vi "Display Contour SPINE Head Tail (SubVI).vi"(0 "Display Data":T1) -> (4 "Contour Array":cluster{"Array":i32[], "Array":i32[]}[](array[cluster]), 6 "SPINE Array":cluster{"Array":i32[], "Array":i32[]}[](array[cluster]), 8 "Head Array":cluster{"Array":i32[], "Array":i32[]}[](array[cluster]), 10 "Tail Array":cluster{"Array":i32[], "Array":i32[]}[](array[cluster]), 15 "Larvae ID":u32[](array[numeric]))   [LabVIEW 2020]
uses:
  Controls (HOST)/Data to Disk Bundle.ctl
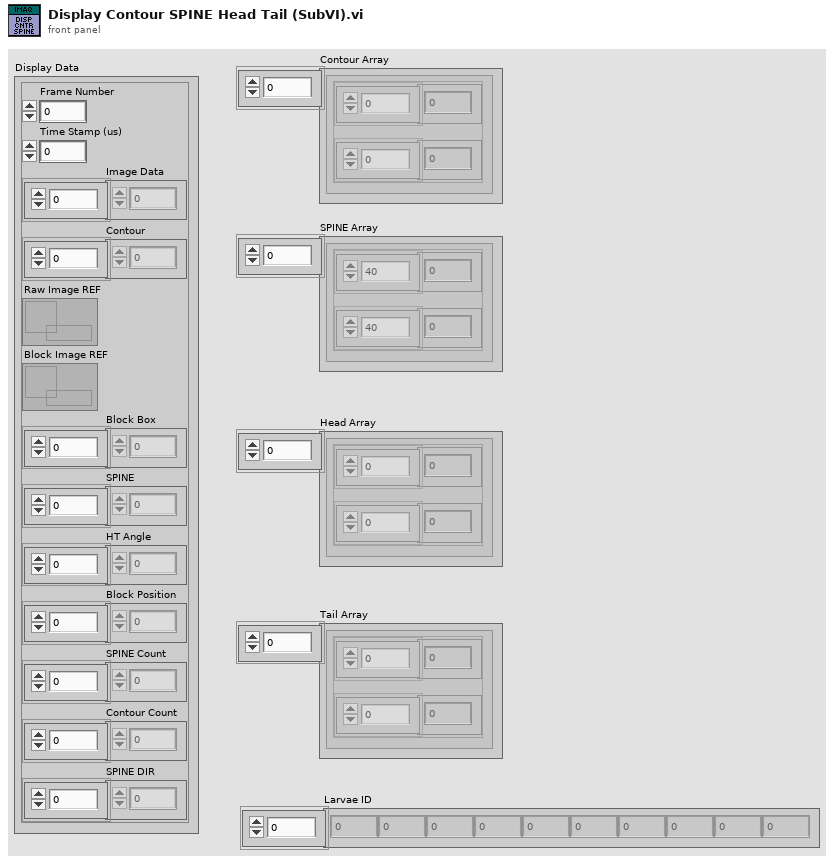
[diagram p1: front panel]
types:
  T1 = typedef "Data to Disk Bundle.ctl" = cluster{"Frame Number":u64, "Time Stamp (us)":u64, "Image Data":u64[], "Contour":u32[], "Raw Image REF":refnum<data-value>, "Block Image REF":refnum<data-value>, "Block Box":u64[], "SPINE":u32[], "HT Angle":u64[], "Block Position":u64[], "SPINE Count":u32[], "Contour Count":u32[], "SPINE DIR":u8[]}
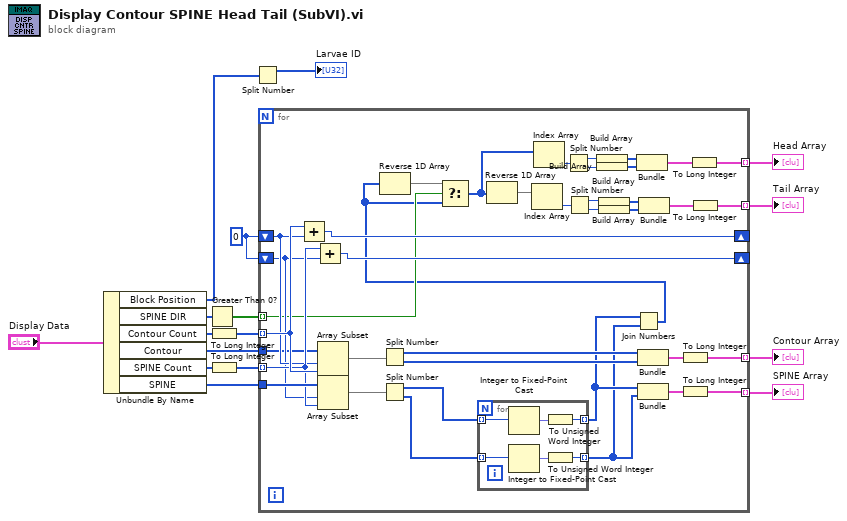
[diagram p0: block diagram]
diagram:
  w14 = 0 ("Numeric Control")
  n1 = Unbundle By Name("Display Data") -> ("Block Position"=w1:u64[], "SPINE DIR"=w3:u8[], "Contour Count"=w9:u32[], "Contour"=w8:u32[], "SPINE Count"=w16:u32[], "SPINE"=w15:u32[])
  n2 = Greater Than 0?(x=w3) -> (x > 0?=w2:bool[])
  n3 = To Long Integer(number=w9) -> (32bit integer=w13:i32[])
  n4 = To Long Integer(number=w16) -> (32bit integer=w12:i32[])
  n5 = Split Number(x=w1) -> (hi(x)=→"Larvae ID":u32[])  [unwired: 1 out]
  n6 = for {
    tunnel: w13 -> [w52] mode=indexing
    tunnel: w8 -> [w39]
    tunnel: w12 -> [w51] mode=indexing
    tunnel: w15 -> [w53]
    shift-right: [w55] -> _
    shift-left: w14 -> [w50]
    shift-right: [w54] -> _
    shift-left: w14 -> [w49]
    tunnel: [w41] -> w10 mode=indexing
    tunnel: [w40] -> w4 mode=indexing
    tunnel: [w25] -> w6 mode=indexing
    tunnel: [w24] -> w5 mode=indexing
    tunnel: w2 -> [w26] mode=indexing
    n7 = Add(x=w52, y=w50) -> (x+y=w55:i32)
    n8 = Add(x=w51, y=w49) -> (x+y=w54:i32)
    n9 = Array Subset(array=w39, index=w50, length=w52) -> (w48:u32[])
    n10 = Array Subset(array=w53, index=w49, length=w51) -> (w27:u32[])
    n11 = Split Number(x=w48) -> (hi(x)=w23:u16[], lo(x)=w22:u16[])
    n12 = Split Number(x=w27) -> (hi(x)=w21:u16[], lo(x)=w20:u16[])
    n13 = for {
      tunnel: w21 -> [w61] mode=indexing
      tunnel: w20 -> [w60] mode=indexing
      tunnel: [w57] -> w19 mode=indexing
      tunnel: [w56] -> w18 mode=indexing
      n14 = Integer to Fixed-Point Cast(integer=w61) -> (fixed-point=w59:fxp<+,16,9>)  [unwired: 1 in]
      n15 = Integer to Fixed-Point Cast(integer=w60) -> (fixed-point=w58:fxp<+,16,9>)  [unwired: 1 in]
      n16 = To Unsigned Word Integer(number=w59) -> (unsigned 16bit integer=w57:u16)
      n17 = To Unsigned Word Integer(number=w58) -> (unsigned 16bit integer=w56:u16)
    }
    n18 = Join Numbers(hi=w19, lo=w18) -> ((hi.lo)=w17:u32[])
    n19 = Reverse 1D Array(array=w17) -> (reversed array=w35:u32[])
    n20 = Select(t=w35, s=w26, f=w17) -> (s? t:f=w36:u32[])
    n21 = Reverse 1D Array(array=w36) -> (reversed array=w32:u32[])
    n22 = Index Array(array=w32) -> (element=w33:u32)  [unwired: 1 in]
    n23 = Index Array(array=w36) -> (element=w34:u32)  [unwired: 1 in]
    n24 = Split Number(x=w34) -> (hi(x)=w28:u16, lo(x)=w29:u16)
    n25 = Split Number(x=w33) -> (hi(x)=w30:u16, lo(x)=w31:u16)
    n26 = Build Array(w28) -> (w45:u16[])
    n27 = Build Array(w29) -> (w44:u16[])
    n28 = Build Array(w30) -> (w42:u16[])
    n29 = Build Array(w31) -> (w43:u16[])
    n30 = Bundle(w45, w44) -> (w37:cluster{u16[], u16[]})  [unwired: 1 in]
    n31 = Bundle(w23, w22) -> (w47:cluster{u16[], u16[]})  [unwired: 1 in]
    n32 = Bundle(w19, w18) -> (w46:cluster{u16[], u16[]})  [unwired: 1 in]
    n33 = Bundle(w42, w43) -> (w38:cluster{u16[], u16[]})  [unwired: 1 in]
    n34 = To Long Integer(number=w47) -> (32bit integer=w41:cluster{i32[], i32[]})
    n35 = To Long Integer(number=w46) -> (32bit integer=w40:cluster{i32[], i32[]})
    n36 = To Long Integer(number=w37) -> (32bit integer=w25:cluster{i32[], i32[]})
    n37 = To Long Integer(number=w38) -> (32bit integer=w24:cluster{i32[], i32[]})
  }
  "Contour Array" <- w10
  "SPINE Array" <- w4
  "Head Array" <- w6
  "Tail Array" <- w5
